vi "OrientationGrip.vi"(8 "error in":errorcluster) -> (0 "error out":errorcluster)   [LabVIEW 2017]
uses:
  Projekt-RubikLibrary/ServoEnumControl.ctl
  Projekt-RubikLibrary/RubikLibrary.lvlib
panel:
  # "Grip from cube left and right\nDon't wait to complete\n\nUse VI in Orientation State Machine"
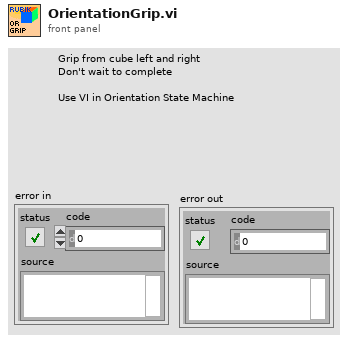
[diagram p1: front panel]
types:
  T1 = typedef "RubikLibrary.lvlib/ServoEnumControl.ctl" = enum16{"Left Servo", "Front Servo", "Right Servo"}
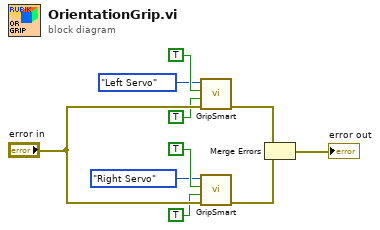
[diagram p0: block diagram]
diagram:
  n1 = call "GripSmart.vi"("error in"="error in", "NoWait"=TRUE ("Turn to (in)"), "Grip closed (in)"=TRUE ("Turn to (in)"), "Servo"=ServoEnumControl."Left Servo") -> ("error out"=w2:errorcluster)  [unwired: 6 in, 1 out]
  n2 = call "GripSmart.vi"("error in"="error in", "NoWait"=TRUE ("Turn to (in)"), "Grip closed (in)"=TRUE, "Servo"=ServoEnumControl."Right Servo") -> ("error out"=w1:errorcluster)  [unwired: 6 in, 1 out]
  n3 = Merge Errors(w2, w1) -> (→"error out":errorcluster)
